vi "iTC_Readout.vi"() -> ()   [LabVIEW 2009]
panel:
  out "millisecond timer value":u32
  out "CCS Resistance":dynamicdata(graph)
  out "Cernox Temperature":dbl(slide) scale=0.0..350.0
  in  "Samples Per Second 6":dbl=15.0
  out "Cernox Temperature":string
  out "Cernox Resistance":dbl(knob) scale=0.0..500.0
  out "Cernox Resistance":string
  out "Cernox Temperature":dynamicdata(graph)
  in  "Samples Per Second 5":dbl=15.0
  out "Allen Bradley Temperature":dbl(slide) scale=0.0..500.0
  out "Allen Bradley Temperature":string
  out "Allen Bradley Temperature":dynamicdata(graph)
  in  "Samples Per Second 4":dbl=15.0
  out "Allen Bradley Resistance":dbl(knob) scale=0.3..300.0
  out "Allen Bradley Resistance":string
  out "Allen Bradley Resistance":dynamicdata(graph)
  in  "Samples Per Second 3":dbl=15.0
  in  "Samples Per Second 2":dbl=15.0
  in  "Samples Per Second":dbl=15.0
  out "CCS Temp":string
  out "CCS Temperature":dynamicdata(graph)
  out "CCS Temp":dbl(slide) scale=0.0..320.0
  out "CCS Resistance":dynamicdata(graph)
  out "CCS Resistance":dbl(knob) scale=0.0..1000.0
  out "CCS Resistance":string
  in  "stop":bool
  out "Measurement":bool caption="Taken"
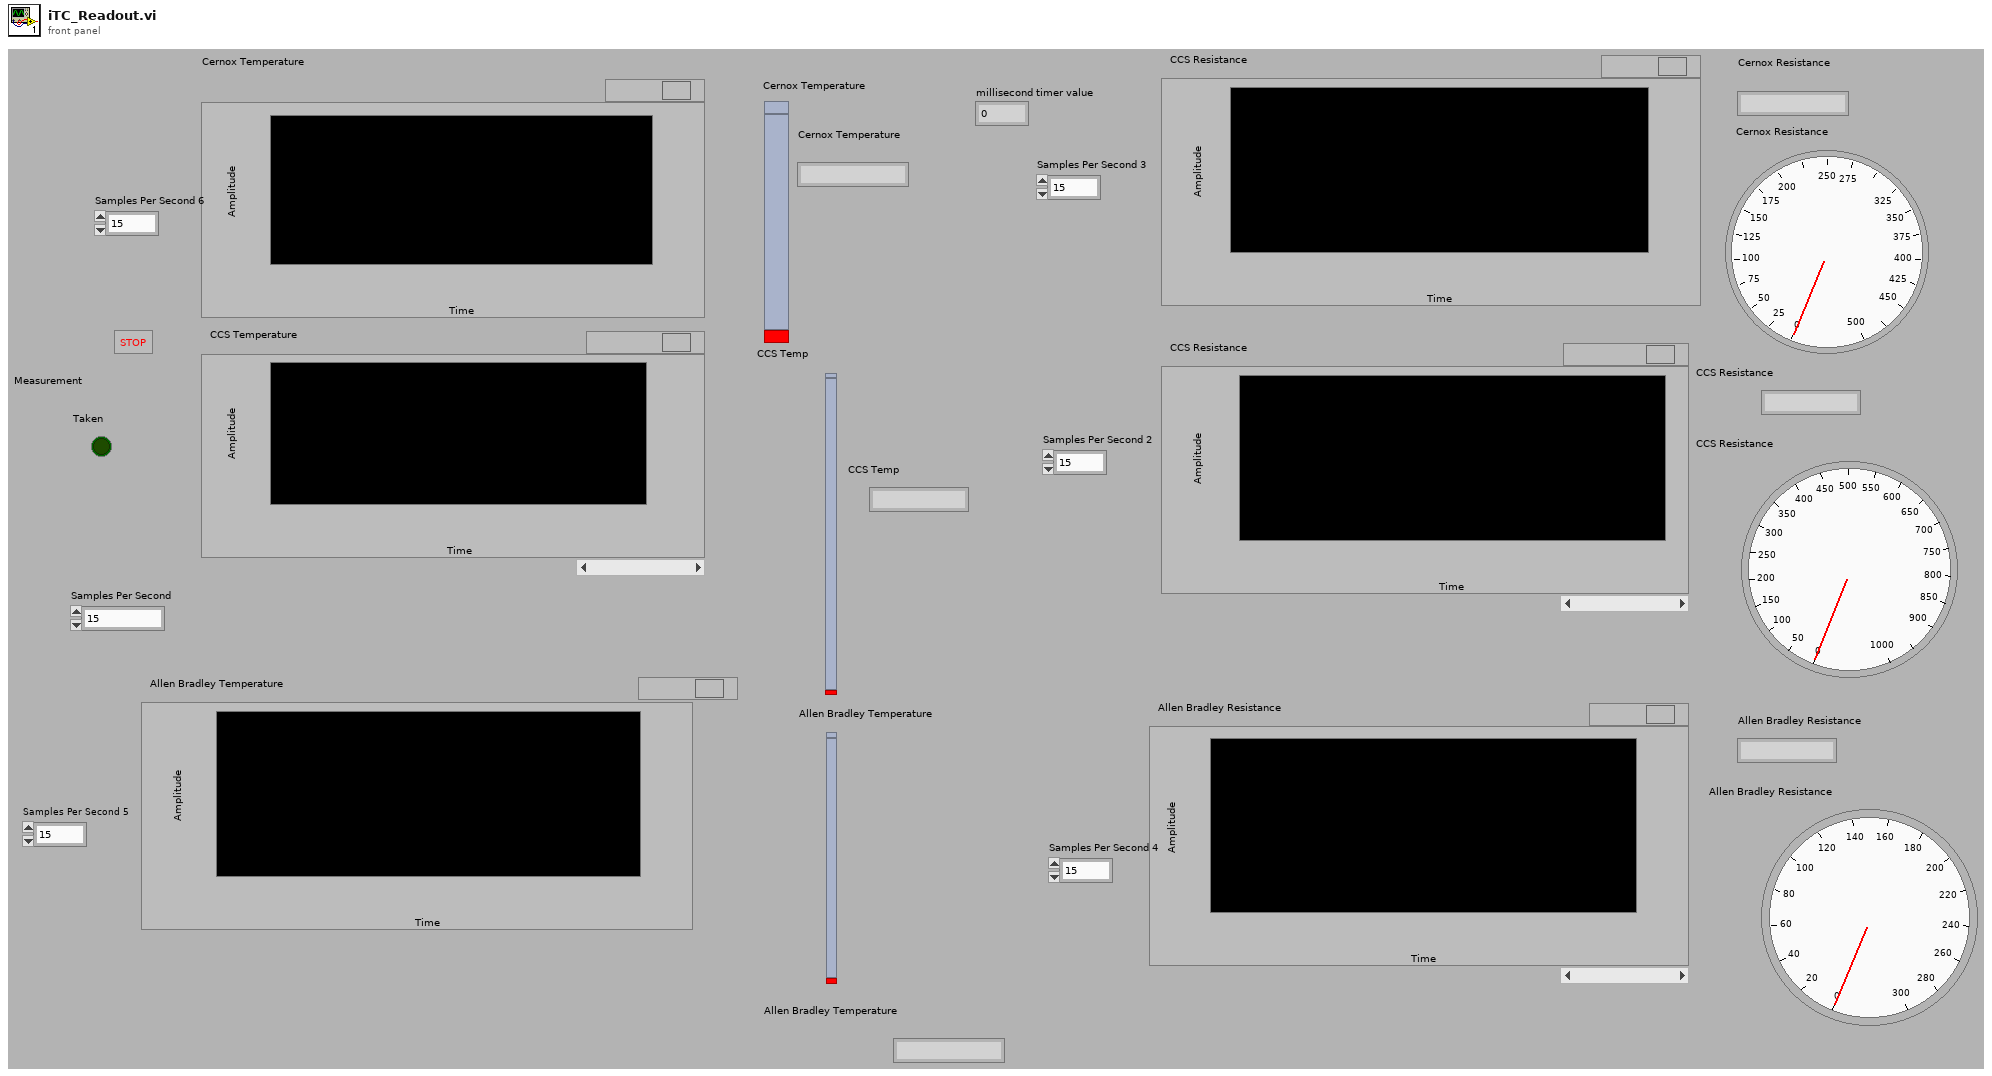
[diagram p1: front panel]
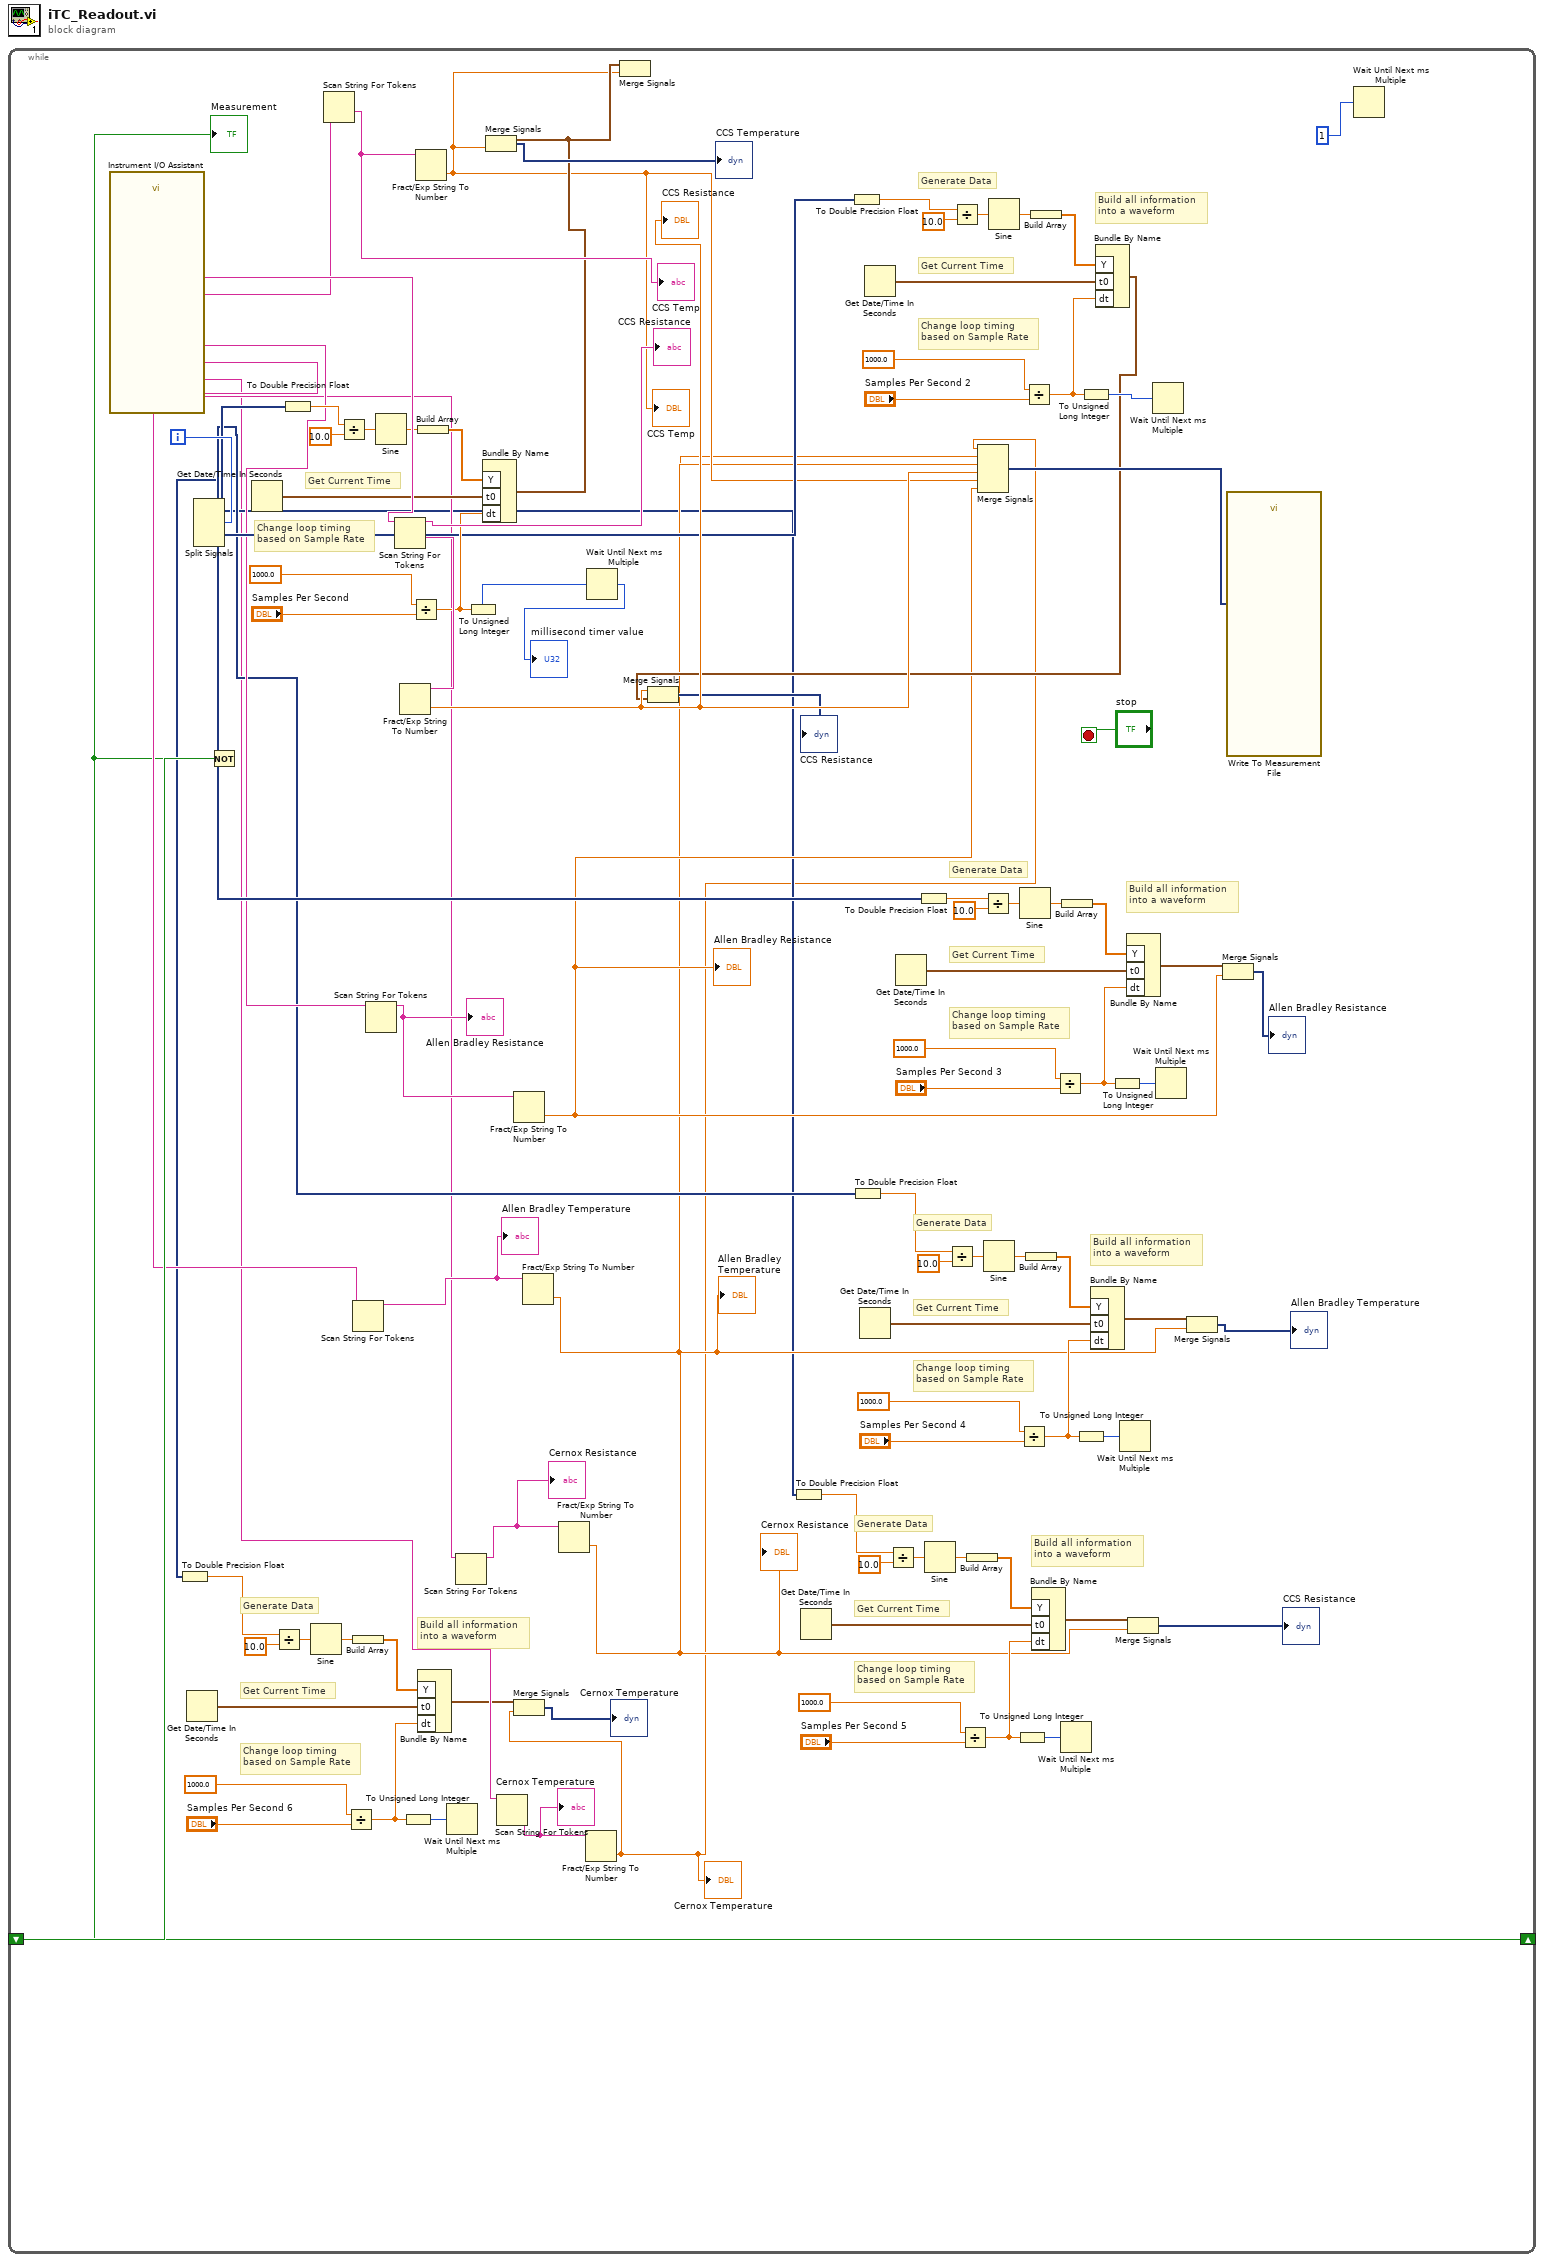
[diagram p0: block diagram]
diagram:
  n1 = while {
    shift-right: [w1] -> _
    shift-left: _ -> [w104]
    i -> [w72]
    stop <- "stop" stop-if-true
    # "Build all information\ninto a waveform"
    # "Change loop timing\nbased on Sample Rate"
    # "Get Current Time"
    # "Generate Data"
    # "Build all information\ninto a waveform"
    # "Change loop timing\nbased on Sample Rate"
    # "Get Current Time"
    # "Generate Data"
    # "Build all information\ninto a waveform"
    # "Change loop timing\nbased on Sample Rate"
    # "Get Current Time"
    # "Generate Data"
    # "Build all information\ninto a waveform"
    # "Change loop timing\nbased on Sample Rate"
    # "Get Current Time"
    # "Generate Data"
    # "Build all information\ninto a waveform"
    # "Change loop timing\nbased on Sample Rate"
    # "Get Current Time"
    # "Generate Data"
    # "Change loop timing\nbased on Sample Rate"
    # "Get Current Time"
    n2 = call "Instrument I/O Assistant"() -> ("token"=w24:string, "CCS Temperature"=w20:string, "Allen Bradley Temperature"=w39:string, "Allen Bradley Resistance"=w55:string, "Cernox Temp"=w100:string, "Cernox Resistance"=w102:string)  [unwired: 21 in, 1 out]
    n3 = Get Date/Time In Seconds() -> (seconds since 1Jan1904=w17:timestamp)
    n4 = Split Signals(w72) -> (w6:dynamicdata, w22:dynamicdata, w37:dynamicdata, w71:dynamicdata, w70:dynamicdata, w57:dynamicdata)  [unwired: 6 in]
    n5 = To Double Precision Float(number=w6) -> (double precision float=w12:dbl)
    n6 = Not(x=w104) -> (.not. x?=w1:bool)
    "Measurement" <- w1
    n7 = Get Date/Time In Seconds() -> (seconds since 1Jan1904=w87:timestamp)
    n8 = Divide(x=w12, y=10.0) -> (x/y=w9:dbl)
    n9 = To Double Precision Float(number=w71) -> (double precision float=w92:dbl)
    n10 = Sine(x=w9) -> (sin(x)=w15:dbl)
    n11 = Scan String For Tokens(9:w100) -> (1:w98:string)  [unwired: 5 in, 3 out]
    "CCS Temp" <- w98
    n12 = Divide(x=w92, y=10.0) -> (x/y=w95:dbl)
    n13 = Divide(x=1000.0, y="Samples Per Second 6") -> (x/y=w18:dbl)
    n14 = Scan String For Tokens(9:w39) -> (3:w38:string)  [unwired: 5 in, 3 out]
    "Allen Bradley Temperature" <- w38
    n15 = Build Array(w15) -> (w16:dbl[])
    n16 = Scan String For Tokens(9:w55) -> (3:w53:string)  [unwired: 5 in, 3 out]
    "Allen Bradley Resistance" <- w53
    n17 = Sine(x=w95) -> (sin(x)=w89:dbl)
    n18 = Scan String For Tokens(9:w102) -> (1:w101:string, 3:→"CCS Resistance":string)  [unwired: 5 in, 2 out]
    n19 = Fract/Exp String To Number(string=w101) -> (number=w75:dbl)  [unwired: 3 in, 1 out]
    "CCS Resistance" <- w75
    n20 = To Unsigned Long Integer(number=w18) -> (unsigned 32bit integer=w11:u32)
    n21 = Divide(x=1000.0, y="Samples Per Second") -> (x/y=w86:dbl)
    n22 = Fract/Exp String To Number(string=w98) -> (number=w68:dbl)  [unwired: 3 in, 1 out]
    "CCS Temp" <- w68
    n23 = Build Array(w89) -> (w88:dbl[])
    n24 = Bundle By Name("Y"=w16, "t0"=w17, "dt"=w18) -> (w8:waveform(dbl))  [unwired: 1 in]
    n25 = Wait Until Next ms Multiple(millisecond multiple=w11) -> ()  [unwired: 1 out]
    n26 = Scan String For Tokens(9:w24) -> (3:w23:string)  [unwired: 5 in, 3 out]
    "Cernox Resistance" <- w23
    n27 = To Unsigned Long Integer(number=w86) -> (unsigned 32bit integer=w93:u32)
    n28 = Bundle By Name("Y"=w88, "t0"=w87, "dt"=w86) -> (w69:waveform(dbl))  [unwired: 1 in]
    n29 = Merge Signals(w69, w68) -> (→"CCS Temperature":dynamicdata)
    n30 = Scan String For Tokens(9:w20) -> (3:w19:string)  [unwired: 5 in, 3 out]
    "Cernox Temperature" <- w19
    n31 = Fract/Exp String To Number(string=w53) -> (number=w52:dbl)  [unwired: 3 in, 1 out]
    "Allen Bradley Resistance" <- w52
    n32 = Fract/Exp String To Number(string=w38) -> (number=w36:dbl)  [unwired: 3 in, 1 out]
    "Allen Bradley Temperature" <- w36
    n33 = Fract/Exp String To Number(string=w23) -> (number=w21:dbl)  [unwired: 3 in, 1 out]
    "Cernox Resistance" <- w21
    n34 = Fract/Exp String To Number(string=w19) -> (number=w5:dbl)  [unwired: 3 in, 1 out]
    "Cernox Temperature" <- w5
    n35 = Merge Signals(w8, w5) -> (→"Cernox Temperature":dynamicdata)
    n36 = Wait Until Next ms Multiple(millisecond multiple=w93) -> (millisecond timer value=→"millisecond timer value":u32)
    n37 = Merge Signals(w69, w68) -> ()  [unwired: 1 out]
    n38 = To Double Precision Float(number=w22) -> (double precision float=w29:dbl)
    n39 = Get Date/Time In Seconds() -> (seconds since 1Jan1904=w34:timestamp)
    n40 = To Double Precision Float(number=w70) -> (double precision float=w79:dbl)
    n41 = To Double Precision Float(number=w37) -> (double precision float=w45:dbl)
    n42 = Get Date/Time In Seconds() -> (seconds since 1Jan1904=w50:timestamp)
    n43 = Get Date/Time In Seconds() -> (seconds since 1Jan1904=w84:timestamp)
    n44 = Divide(x=w29, y=10.0) -> (x/y=w26:dbl)
    n45 = Get Date/Time In Seconds() -> (seconds since 1Jan1904=w66:timestamp)
    n46 = To Double Precision Float(number=w57) -> (double precision float=w61:dbl)
    n47 = Sine(x=w26) -> (sin(x)=w32:dbl)
    n48 = Divide(x=w45, y=10.0) -> (x/y=w42:dbl)
    n49 = Divide(x=w79, y=10.0) -> (x/y=w76:dbl)
    n50 = Divide(x=1000.0, y="Samples Per Second 5") -> (x/y=w35:dbl)
    n51 = Build Array(w32) -> (w33:dbl[])
    n52 = Merge Signals(w5, w21, w36, w75, w68, w52) -> (w99:dynamicdata)
    n53 = Divide(x=w61, y=10.0) -> (x/y=w58:dbl)
    n54 = Sine(x=w42) -> (sin(x)=w48:dbl)
    n55 = Sine(x=w76) -> (sin(x)=w82:dbl)
    n56 = To Unsigned Long Integer(number=w35) -> (unsigned 32bit integer=w28:u32)
    n57 = Divide(x=1000.0, y="Samples Per Second 4") -> (x/y=w51:dbl)
    n58 = Sine(x=w58) -> (sin(x)=w64:dbl)
    n59 = Divide(x=1000.0, y="Samples Per Second 2") -> (x/y=w85:dbl)
    n60 = Build Array(w48) -> (w49:dbl[])
    n61 = Build Array(w82) -> (w83:dbl[])
    n62 = Bundle By Name("Y"=w33, "t0"=w34, "dt"=w35) -> (w25:waveform(dbl))  [unwired: 1 in]
    n63 = Divide(x=1000.0, y="Samples Per Second 3") -> (x/y=w67:dbl)
    n64 = Wait Until Next ms Multiple(millisecond multiple=w28) -> ()  [unwired: 1 out]
    n65 = Build Array(w64) -> (w65:dbl[])
    n66 = To Unsigned Long Integer(number=w51) -> (unsigned 32bit integer=w44:u32)
    n67 = To Unsigned Long Integer(number=w85) -> (unsigned 32bit integer=w78:u32)
    n68 = Bundle By Name("Y"=w49, "t0"=w50, "dt"=w51) -> (w41:waveform(dbl))  [unwired: 1 in]
    n69 = Bundle By Name("Y"=w83, "t0"=w84, "dt"=w85) -> (w73:waveform(dbl))  [unwired: 1 in]
    n70 = Merge Signals(w75, w73) -> (→"CCS Resistance":dynamicdata)
    n71 = To Unsigned Long Integer(number=w67) -> (unsigned 32bit integer=w60:u32)
    n72 = Wait Until Next ms Multiple(millisecond multiple=w44) -> ()  [unwired: 1 out]
    n73 = Bundle By Name("Y"=w65, "t0"=w66, "dt"=w67) -> (w56:waveform(dbl))  [unwired: 1 in]
    n74 = Merge Signals(w25, w21) -> (→"CCS Resistance":dynamicdata)
    n75 = Wait Until Next ms Multiple(millisecond multiple=w78) -> ()  [unwired: 1 out]
    n76 = Wait Until Next ms Multiple(millisecond multiple=w60) -> ()  [unwired: 1 out]
    n77 = Merge Signals(w41, w36) -> (→"Allen Bradley Temperature":dynamicdata)
    n78 = Merge Signals(w56, w52) -> (→"Allen Bradley Resistance":dynamicdata)
    n79 = call "Write To Measurement File"("Signals"=w99) -> ()  [unwired: 16 in, 3 out]
    n80 = Wait Until Next ms Multiple(millisecond multiple=u32 1) -> ()  [unwired: 1 out]
  }
